vi "SentinelController v35 good v11.vi"() -> ()   [LabVIEW 2011] (continued)
                                n794 = Concatenate Strings(w2879, w2880, w2890, "   " ("string"), w2891, w2880, "H1 Warning, H2 Alarming", w2880, w2899, w2880, "H1 Low Yield Warning Limit: ", w2901, ", H1 yield = ", w2903, w2880, "H1 Low UPH Warning Limit: ", w2905, ", H1 UPH = ", w2907, w2880, w2908, w2880, "H2 Low Yield Alarm Limit: ", w2910, ", H2 yield = ", w2912, w2880, "H2 Low UPH Alarm Limit: ", w2914, ", H2 UPH = ", w2916, w2880, w2880) -> (w2888:string)
                                n795 = call "SentinelDatalog.vi"("operation (0:open)"=T10."open", "String"=w2888, "data log path"=w2882) -> ()  [unwired: 8 in, 1 out]
                                }
                                frame "H1AH2N" {
                                w2927 = "\r\n"
                                n796 = local read "H1 online"() -> (w2944:bool)
                                n797 = local read "H2 online"() -> (w2945:bool)
                                n798 = local read "H2 UPH warning limit hid"() -> (w2942:dbl)
                                n799 = local read "H2  low yield warning"() -> (w2941:dbl)
                                n800 = local read "H1 UPH alarm limit hid"() -> (w2940:dbl)
                                n801 = local read "H1 low yield alarm"() -> (w2939:dbl)
                                n802 = local read "H1 UPH"() -> (w2933:cluster{u32, u32})
                                n803 = local read "H2 UPH"() -> (w2932:cluster{u32, u32})
                                n804 = local read "YieldMon"() -> (w2925:cluster{i32, i32, i32, i32})
                                n805 = local read "YieldMon"() -> (w2923:cluster{i32, i32, i32, i32})
                                n806 = case shown="True" w2944 {
                                tunnel: ["H1 Off-Line" "H1 On-Line"] -> w2946
                                frame False {
                                }
                                frame True {
                                }
                                }
                                n807 = case shown="False" w2945 {
                                tunnel: ["H2 Off-Line" "H2 On-Line"] -> w2955
                                frame False {
                                }
                                frame True {
                                }
                                }
                                n808 = local read "Number of data log entries hid"() -> (w2921:u32)
                                n809 = Unbundle(w2925) -> (w2924:i32)  [unwired: 3 out]
                                n810 = Unbundle(w2933) -> (w2931:u32)  [unwired: 1 out]
                                n811 = Unbundle(w2923) -> (w2922:i32)  [unwired: 3 out]
                                n812 = Unbundle(w2932) -> (w2930:u32)  [unwired: 1 out]
                                n813 = Number To Decimal String(number=w2939) -> (decimal integer string=w2948:string)  [unwired: 1 in]
                                n814 = Number To Decimal String(number=w2924) -> (decimal integer string=w2950:string)  [unwired: 1 in]
                                n815 = Number To Decimal String(number=w2940) -> (decimal integer string=w2952:string)  [unwired: 1 in]
                                n816 = Number To Decimal String(number=w2931) -> (decimal integer string=w2954:string)  [unwired: 1 in]
                                n817 = Number To Decimal String(number=w2941) -> (decimal integer string=w2957:string)  [unwired: 1 in]
                                n818 = Number To Decimal String(number=w2922) -> (decimal integer string=w2959:string)  [unwired: 1 in]
                                n819 = Number To Decimal String(number=w2942) -> (decimal integer string=w2961:string)  [unwired: 1 in]
                                n820 = Number To Decimal String(number=w2930) -> (decimal integer string=w2963:string)  [unwired: 1 in]
                                n821 = local read "Data log path and filename"() -> (w2929:path)
                                n822 = Get Date/Time String(want seconds? (F)=TRUE) -> (date string=w2937:string, time string=w2938:string)  [unwired: 2 in]
                                n823 = Number To Decimal String(number=w2921) -> (decimal integer string=w2926:string)  [unwired: 1 in]
                                n824 = Concatenate Strings(w2926, w2927, w2937, "   " ("string"), w2938, w2927, "H1 Alarming, H2 Nominal", w2927, w2946, w2927, "H1 Low Yield Alarm Limit: ", w2948, ", H1 yield = ", w2950, w2927, "H1 Low UPH Alarm Limit: ", w2952, ", H1 UPH = ", w2954, w2927, w2955, w2927, "H2 Low Yield Warning Limit: ", w2957, ", H2 yield = ", w2959, w2927, "H2 Low UPH Warning Limit: ", w2961, ", H2 UPH = ", w2963, w2927, w2927) -> (w2935:string)
                                n825 = call "SentinelDatalog.vi"("operation (0:open)"=T10."open", "String"=w2935, "data log path"=w2929) -> ()  [unwired: 8 in, 1 out]
                                }
                                frame "H1AH2W" {
                                w2974 = "\r\n"
                                n826 = local read "H1 online"() -> (w2991:bool)
                                n827 = local read "H2 online"() -> (w2992:bool)
                                n828 = local read "H2 UPH warning limit hid"() -> (w2989:dbl)
                                n829 = local read "H2  low yield warning"() -> (w2988:dbl)
                                n830 = local read "H1 UPH alarm limit hid"() -> (w2987:dbl)
                                n831 = local read "H1 low yield alarm"() -> (w2986:dbl)
                                n832 = local read "H1 UPH"() -> (w2980:cluster{u32, u32})
                                n833 = local read "H2 UPH"() -> (w2979:cluster{u32, u32})
                                n834 = local read "YieldMon"() -> (w2972:cluster{i32, i32, i32, i32})
                                n835 = local read "YieldMon"() -> (w2970:cluster{i32, i32, i32, i32})
                                n836 = case shown="True" w2991 {
                                tunnel: ["H1 Off-Line" "H1 On-Line"] -> w2993
                                frame False {
                                }
                                frame True {
                                }
                                }
                                n837 = case shown="True" w2992 {
                                tunnel: ["H2 Off-Line" "H2 On-Line"] -> w3002
                                frame False {
                                }
                                frame True {
                                }
                                }
                                n838 = local read "Number of data log entries hid"() -> (w2968:u32)
                                n839 = Unbundle(w2972) -> (w2971:i32)  [unwired: 3 out]
                                n840 = Unbundle(w2980) -> (w2978:u32)  [unwired: 1 out]
                                n841 = Unbundle(w2970) -> (w2969:i32)  [unwired: 3 out]
                                n842 = Unbundle(w2979) -> (w2977:u32)  [unwired: 1 out]
                                n843 = Number To Decimal String(number=w2986) -> (decimal integer string=w2995:string)  [unwired: 1 in]
                                n844 = Number To Decimal String(number=w2971) -> (decimal integer string=w2997:string)  [unwired: 1 in]
                                n845 = Number To Decimal String(number=w2987) -> (decimal integer string=w2999:string)  [unwired: 1 in]
                                n846 = Number To Decimal String(number=w2978) -> (decimal integer string=w3001:string)  [unwired: 1 in]
                                n847 = Number To Decimal String(number=w2988) -> (decimal integer string=w3004:string)  [unwired: 1 in]
                                n848 = Number To Decimal String(number=w2969) -> (decimal integer string=w3006:string)  [unwired: 1 in]
                                n849 = Number To Decimal String(number=w2989) -> (decimal integer string=w3008:string)  [unwired: 1 in]
                                n850 = Number To Decimal String(number=w2977) -> (decimal integer string=w3010:string)  [unwired: 1 in]
                                n851 = local read "Data log path and filename"() -> (w2976:path)
                                n852 = Get Date/Time String(want seconds? (F)=TRUE) -> (date string=w2984:string, time string=w2985:string)  [unwired: 2 in]
                                n853 = Number To Decimal String(number=w2968) -> (decimal integer string=w2973:string)  [unwired: 1 in]
                                n854 = Concatenate Strings(w2973, w2974, w2984, "   " ("string"), w2985, w2974, "H1 Alarming, H2 Warning", w2974, w2993, w2974, "H1 Low Yield Alarm Limit: ", w2995, ", H1 yield = ", w2997, w2974, "H1 Low UPH Alarm Limit: ", w2999, ", H1 UPH = ", w3001, w2974, w3002, w2974, "H2 Low Yield Warning Limit: ", w3004, ", H2 yield = ", w3006, w2974, "H2 Low UPH Warning Limit: ", w3008, ", H2 UPH = ", w3010, w2974) -> (w2982:string)
                                n855 = call "SentinelDatalog.vi"("operation (0:open)"=T10."open", "String"=w2982, "data log path"=w2976) -> ()  [unwired: 8 in, 1 out]
                                }
                                frame "H1AH2A" {
                                w3021 = "\r\n"
                                n856 = local read "H1 online"() -> (w3038:bool)
                                n857 = local read "H2 online"() -> (w3039:bool)
                                n858 = local read "H1 UPH alarm limit hid"() -> (w3034:dbl)
                                n859 = local read "H2 UPH alarm limit hid"() -> (w3036:dbl)
                                n860 = local read "H1 low yield alarm"() -> (w3033:dbl)
                                n861 = local read "H1 UPH"() -> (w3027:cluster{u32, u32})
                                n862 = local read "H2 low yield alarm"() -> (w3035:dbl)
                                n863 = local read "H2 UPH"() -> (w3026:cluster{u32, u32})
                                n864 = local read "YieldMon"() -> (w3019:cluster{i32, i32, i32, i32})
                                n865 = local read "YieldMon"() -> (w3018:cluster{i32, i32, i32, i32})
                                n866 = case shown="True" w3038 {
                                tunnel: ["H1 Off-Line" "H1 On-Line"] -> w3040
                                frame False {
                                }
                                frame True {
                                }
                                }
                                n867 = case shown="True" w3039 {
                                tunnel: ["H2 Off-Line" "H2 On-Line"] -> w3049
                                frame False {
                                }
                                frame True {
                                }
                                }
                                n868 = local read "Number of data log entries hid"() -> (w3015:u32)
                                n869 = Unbundle(w3019) -> (w3016:i32)  [unwired: 3 out]
                                n870 = Unbundle(w3027) -> (w3025:u32)  [unwired: 1 out]
                                n871 = Unbundle(w3018) -> (w3017:i32)  [unwired: 3 out]
                                n872 = Unbundle(w3026) -> (w3024:u32)  [unwired: 1 out]
                                n873 = Number To Decimal String(number=w3033) -> (decimal integer string=w3042:string)  [unwired: 1 in]
                                n874 = Number To Decimal String(number=w3016) -> (decimal integer string=w3044:string)  [unwired: 1 in]
                                n875 = Number To Decimal String(number=w3034) -> (decimal integer string=w3046:string)  [unwired: 1 in]
                                n876 = Number To Decimal String(number=w3025) -> (decimal integer string=w3048:string)  [unwired: 1 in]
                                n877 = Number To Decimal String(number=w3035) -> (decimal integer string=w3051:string)  [unwired: 1 in]
                                n878 = Number To Decimal String(number=w3017) -> (decimal integer string=w3053:string)  [unwired: 1 in]
                                n879 = Number To Decimal String(number=w3036) -> (decimal integer string=w3055:string)  [unwired: 1 in]
                                n880 = Number To Decimal String(number=w3024) -> (decimal integer string=w3057:string)  [unwired: 1 in]
                                n881 = local read "Data log path and filename"() -> (w3023:path)
                                n882 = Get Date/Time String(want seconds? (F)=TRUE) -> (date string=w3031:string, time string=w3032:string)  [unwired: 2 in]
                                n883 = Number To Decimal String(number=w3015) -> (decimal integer string=w3020:string)  [unwired: 1 in]
                                n884 = Concatenate Strings(w3020, w3021, w3031, "   " ("string"), w3032, w3021, "H1 Alarming, H2 Alarming", w3021, w3040, w3021, "H1 Low Yield Alarm Limit: ", w3042, ", H1 yield = ", w3044, w3021, "H1 Low UPH Alarm Limit: ", w3046, ", H1 UPH = ", w3048, w3021, w3049, w3021, "H2 Low Yield Alarm Limit: ", w3051, ", H2 yield = ", w3053, w3021, "H2 Low UPH Alarm Limit: ", w3055, ", H2 UPH = ", w3057, w3021, w3021) -> (w3029:string)
                                n885 = call "SentinelDatalog.vi"("operation (0:open)"=T10."open", "String"=w3029, "data log path"=w3023) -> ()  [unwired: 8 in, 1 out]
                                }
                                }
                                }
                                frame #2 {
                                n886 = Wait (ms)(milliseconds to wait=u32 100) -> ()  [unwired: 1 out]
                                }
                                frame #3 {
                                n887 = local read "Enable electronic notification of alarms"() -> (w3063:bool)
                                n888 = case shown="True" w3063 {
                                frame False {
                                }
                                frame True {
                                n889 = stacked-sequence {
                                frame #0 {
                                # "Email"
                                n890 = local read "Enable email notification"() -> (w3066:bool)
                                n891 = local read "Number of email alerts"() -> (w3065:u32)
                                n892 = Increment(x=w3065) -> (x+1=w3064:u32)
                                n893 = local write "Number of email alerts"(w3064) -> ()
                                n894 = case shown="True" w3066 {
                                frame False {
                                }
                                frame True {
                                n895 = flat-sequence {
                                tunnel: [w3073] -> w3068
                                tunnel: [w3081] -> w3067
                                tunnel: w3068 -> [w3081]
                                tunnel: w3067 -> [w3082]
                                frame #0 {
                                n896 = local read "Data log path and filename"() -> (w3078:path)
                                n897 = local read "Number of email alerts"() -> (w3072:u32)
                                n898 = Number To Decimal String(number=w3072) -> (decimal integer string=w3071:string)  [unwired: 1 in]
                                n899 = Strip Path(path=w3078) -> (stripped path=w3076:path, name=w3070:string)
                                n900 = Path To String(path=w3076) -> (string=w3075:string)
                                n901 = Concatenate Strings(w3075, "\\sent_#" ("string"), w3071, "_" ("string"), w3070) -> (w3079:string)
                                n902 = String To Path(string=w3079) -> (path=w3074:path)
                                n903 = Copy(10:w3074, 11:w3078) -> (3:w3073:path)  [unwired: 3 in, 2 out]
                                }
                                frame #1 {
                                n904 = Wait (ms)(milliseconds to wait=u32 1000) -> ()  [unwired: 1 out]
                                }
                                frame #2 {
                                n905 = local read "Email alert - engineer"() -> (w3084:string)
                                n906 = local read "Email alert - CC"() -> (w3083:string)
                                n907 = local read "Email alert - message"() -> (w3085:string)
                                n908 = call "email_alert.vi"("Email Alert - Message"=w3085, "Email Alert - Engineer"=w3084, "Email Alert - CC"=w3083, "Email ALert - Attachment"=w3082) -> ()  [unwired: 8 in]
                                }
                                }
                                }
                                }
                                }
                                frame #1 {
                                n909 = Wait (ms)(milliseconds to wait=u32 200) -> ()  [unwired: 1 out]
                                }
                                frame #2 {
                                # "text"
                                n910 = local read "Enable text notification"() -> (w3087:bool)
                                n911 = case shown="True" w3087 {
                                frame False {
                                }
                                frame True {
                                n912 = local read "Number of text alerts"() -> (w3091:u32)
                                n913 = Increment(x=w3091) -> (x+1=w3090:u32)
                                n914 = local write "Number of text alerts"(w3090) -> ()
                                n915 = local read "Number of email alerts"() -> (w3100:u32)
                                n916 = local read "Carrier"() -> (w3093:enum16{"T-Mobile", "AT&T", "Verizon", "Sprint"})
                                n917 = local read "Phone number"() -> (w3092:string)
                                n918 = local read "Body"() -> (w3089:string)
                                n919 = local read "Lot number"() -> (w3094:string)
                                n920 = local read "Subject"() -> (w3088:string)
                                n921 = Number To Decimal String(number=w3100) -> (decimal integer string=w3096:string)  [unwired: 1 in]
                                n922 = Concatenate Strings(w3089, ", # " ("string"), w3096, ", Lot Number: " ("string"), w3094) -> (w3101:string)
                                n923 = local write "Notifications Lot Display"(w3094) -> ()
                                n924 = call <userlib>:"Send SMS 2009.vi"("Body"=w3101, "Carrier"=w3093, "Subject"=w3088, "phone number"=w3092, "smtp server"="smtp.gmail.com", "password"="sentinelcontroller", "email username"="sentinelcontroller@gmail.com") -> ("Error Out"=w3099:errorcluster)  [unwired: 4 in]
                                n925 = Unbundle By Name(w3099) -> ("status"=w3098:bool)
                                n926 = case shown="True" w3098 {
                                frame False {
                                }
                                frame True {
                                n927 = One Button Dialog(message="Warning:\nError sending text message!\nTry changing the settings or\nswitch to email method", button name ("OK")="Dismiss") -> ()  [unwired: 1 out]
                                }
                                }
                                }
                                }
                                }
                                }
                                }
                                }
                                }
                                frame #4 {
                                n928 = Wait (ms)(milliseconds to wait=u32 100) -> ()  [unwired: 1 out]
                                }
                              }
                            }
                          }
                        }
                      }
                    }
                  }
                }
              }
              n929 = Wait (ms)(milliseconds to wait=u32 100) -> ()  [unwired: 1 out]
            }
            n930 = local read "Yield averaging"() -> (w350:u32)
            n931 = local read "UPH averaging"() -> (w349:u32)
            n932 = local read "Yield averaging"() -> (w351:u32)
            n933 = local read "UPH averaging"() -> (w352:u32)
            n934 = Initialize Array(w347, w350) -> (w348:i32[])
            n935 = Initialize Array(w346, w349) -> (w345:dbl[])
            n936 = Initialize Array(w354, w351) -> (w353:i32[])
            n937 = Initialize Array(w355, w352) -> (w356:dbl[])
            n938 = while {
              shift-right: [w2370] -> _
              shift-left: w346 -> [w2376]
              shift-right: [w2371] -> _
              shift-left: w345 -> [w2375]
              shift-right: [w2372] -> _
              shift-left: w347 -> [w2369]
              shift-right: [w2373] -> _
              shift-left: w348 -> [w2374]
              stop <- w2367 stop-if-true
              # "if there is now a lock, it is unlikely that the test time is going to be less than 100ms,\nso this is a relatively slow loop"
              n939 = local read "H2 Lock"() -> (w2366:bool)
              n940 = Wait (ms)(milliseconds to wait=u32 50) -> ()  [unwired: 1 out]
              n941 = case shown="True" w2366 {
                tunnel: w2376 -> [w2381 w2406]
                tunnel: w2375 -> [w2380 w2401]
                tunnel: w2374 -> [w2378 w2398]
                tunnel: [w2378 w2392] -> w2373
                tunnel: [w2379 w2390] -> w2372
                tunnel: [w2380 w2389] -> w2371
                tunnel: [w2381 w2388] -> w2370
                tunnel: w2369 -> [w2379 w2387]
                frame False {
                  n942 = local write "Calc H1 UPH"(u32 0 ("Sim H1 UPH")) -> ()
                }
                frame True {
                  n943 = flat-sequence {
                    tunnel: w2398 -> [w2409]
                    tunnel: w2387 -> [w2410]
                    tunnel: w2401 -> [w2411]
                    tunnel: w2406 -> [w2412]
                    tunnel: [w2412] -> w2397
                    tunnel: [w2411] -> w2396
                    tunnel: [w2410] -> w2395
                    tunnel: [w2409] -> w2394
                    tunnel: [w2425] -> w2405
                    tunnel: [w2424] -> w2402
                    tunnel: [w2423] -> w2400
                    tunnel: [w2422] -> w2399
                    tunnel: w2397 -> [w2425]
                    tunnel: w2396 -> [w2424]
                    tunnel: w2395 -> [w2423]
                    tunnel: w2394 -> [w2422]
                    tunnel: w2405 -> [w2451]
                    tunnel: [w2451] -> w2404
                    tunnel: [w2450] -> w2403
                    tunnel: w2402 -> [w2450]
                    tunnel: w2400 -> [w2440]
                    tunnel: w2399 -> [w2439]
                    tunnel: [w2438] -> w2393
                    tunnel: [w2437] -> w2391
                    tunnel: w2404 -> [w2477]
                    tunnel: w2403 -> [w2478]
                    tunnel: w2393 -> [w2496]
                    tunnel: w2391 -> [w2495]
                    tunnel: [w2496] -> w2386
                    tunnel: [w2495] -> w2385
                    tunnel: [w2474] -> w2384
                    tunnel: [w2473] -> w2383
                    tunnel: [w2511] -> w2388
                    tunnel: [w2512] -> w2389
                    tunnel: [w2513] -> w2390
                    tunnel: [w2514] -> w2392
                    tunnel: w2386 -> [w2514]
                    tunnel: w2385 -> [w2513]
                    tunnel: w2384 -> [w2512]
                    tunnel: w2383 -> [w2511]
                    frame #0 {
                      n944 = local read "H2 loop counter hid"() -> (w2407:u32)
                      n945 = Equal To 0?(x=w2407) -> (x = 0?=w2408:bool)
                      n946 = case shown="True" w2408 {
                        frame False {
                        }
                        frame True {
                          # "H2 first pass init"
                          n947 = local write "H2 Device Count"(0.0 ("H2 Device Count")) -> ()
                          n948 = local write "H2 measured  Index Time"(0.0 ("H2 Index Time")) -> ()
                          n949 = local write "H2 measured Test Time"(0.0 ("H2 Test Time")) -> ()
                          n950 = local write "H2 measured Wait Time"(0.0 ("H2 Wait Time")) -> ()
                          n951 = local read "H2 low UPH alarm (%)"() -> (w2416:dbl)
                          n952 = Divide(x=w2416, y=100.0) -> (x/y=w2415:dbl)
                          n953 = Bundle(0.0, w2415) -> (w2413:cluster{dbl, dbl})  [unwired: 1 in]
                          n954 = local write "H2 UPH"(w2413) -> ()
                        }
                      }
                    }
                    frame #1 {
                      # "H2 testing"
                      n955 = while {
                        stop <- w2429 stop-if-true
                        n956 = local read "H2 Lock"() -> (w2433:bool)
                        n957 = local read "POWER"() -> (w2428:bool)
                        n958 = local read "Run"() -> (w2426:bool)
                        n959 = Not(x=w2433) -> (.not. x?=w2427:bool)
                        n960 = Not(x=w2428) -> (.not. x?=w2431:bool)
                        n961 = Not(x=w2426) -> (.not. x?=w2430:bool)
                        n962 = Compound Arithmetic op=OR(w2427, w2431, w2430) -> (w2429:bool)
                        n963 = Wait (ms)(milliseconds to wait=u32 1) -> ()  [unwired: 1 out]
                      }
                    }
                    frame #2 {
                      n964 = local read "H2 cycle yield hid"() -> (w2434:dbl)
                      n965 = local read "H2 loop counter hid"() -> (w2435:u32)
                      n966 = local read "Yield averaging"() -> (w2436:u32)
                      n967 = local read "H2 low yield alarm"() -> (w2449:dbl)
                      n968 = local read "YieldMon"() -> (w2442:cluster{i32, i32, i32, i32})
                      n969 = local read "H2  low yield warning"() -> (w2448:dbl)
                      n970 = call "moving_avg_core.vi"("Array in"=w2439, "avg"=w2436, "accumulator in"=w2440, "i"=w2435, "data in"=w2434) -> ("Array out"=w2438:dbl[], "accumulator out"=w2437:dbl, "rolling avg out"=w2443:dbl)  [unwired: 4 in]
                      n971 = Unbundle(w2442) -> (w2441:i32)  [unwired: 3 out]
                      n972 = Less?(x=w2443, y=w2448) -> (x < y?=w2447:bool)
                      n973 = case shown="True" w2447 {
                        tunnel: w2443 -> [_ w2456]
                        tunnel: w2449 -> [_ w2455]
                        frame False {
                          n974 = local write "H2 nominal"(TRUE ("H1 nominal")) -> ()
                          n975 = local write "H2 warning"(FALSE ("H1 warning")) -> ()
                          n976 = local write "H2 alarm"(FALSE ("H1 warning")) -> ()
                        }
                        frame True {
                          n977 = Less?(x=w2456, y=w2455) -> (x < y?=w2457:bool)
                          n978 = case shown="True" w2457 {
                            frame False {
                              n979 = local write "H2 nominal"(FALSE ("H1 nominal")) -> ()
                              n980 = local write "H2 warning"(TRUE ("H1 warning")) -> ()
                              n981 = local write "H2 alarm"(FALSE ("H1 warning")) -> ()
                            }
                            frame True {
                              n982 = local read "H2 enable halt\non yield alarm"() -> (w2461:bool)
                              n983 = local write "H2 nominal"(FALSE ("H1 nominal")) -> ()
                              n984 = local write "H2 alarm"(TRUE ("H1 warning")) -> ()
                              n985 = local write "H2 warning"(FALSE ("H1 warning")) -> ()
                              n986 = case shown="True" w2461 {
                                frame False {
                                }
                                frame True {
                                n987 = local write "H2 online"(FALSE ("H1 Online")) -> ()
                                }
                              }
                            }
                          }
                        }
                      }
                      n988 = local read "H1 low yield alarm"() -> (w2446:dbl)
                      n989 = local read "H2 low yield alarm"() -> (w2445:dbl)
                      n990 = Bundle(w2441, "rolling avg out"=w2443, "H1 low yield alarm"=w2446, "H2 low yield alarm"=w2445) -> (w2444:T12)  [unwired: 1 in]
                      n991 = local write "YieldMon"(w2444) -> ()
                    }
                    frame #3 {
                      n992 = local read "H2 measured  Index Time"() -> (w2467:dbl)
                      n993 = local read "H2 measured Wait Time"() -> (w2466:dbl)
                      n994 = local read "H2 measured Test Time"() -> (w2468:dbl)
                      n995 = local read "H2 parallelism"() -> (w2480:u32)
                      n996 = local read "H2 lot yield mon"() -> (w2494:dbl)
                      n997 = local write "H2 IT (scycle)"(w2467) -> ()
                      n998 = local write "H2 TT (s/cycle)"(w2468) -> ()
                      n999 = local write "H2 WT (s/cycle)"(w2466) -> ()
                      n1000 = Compound Arithmetic op=ADD(w2467, w2468, w2466) -> (w2483:dbl)
                      n1001 = Compound Arithmetic op=ADD(w2467, w2468) -> (w2479:dbl)
                      n1002 = Multiply(x=w2480, y=3600.0 ("x")) -> (x*y=w2482:dbl)
                      n1003 = Divide(x=w2482, y=w2483) -> (x/y=w2493:dbl)
                      n1004 = Divide(x=w2494, y=w2479) -> (x/y=w2472:dbl)
                      n1005 = local write "H2 Single Handler UPH hid"(w2472) -> ()
                      n1006 = local read "H2 low UPH warning (%)"() -> (w2490:dbl)
                      n1007 = local read "H2 loop counter hid"() -> (w2476:u32)
                      n1008 = local read "Yield averaging"() -> (w2475:u32)
                      n1009 = local read "H2 low UPH alarm (%)"() -> (w2485:dbl)
                      n1010 = property on="H2 UPH" class="Knob (strict)"() -> ("Scale.Maximum"=w2491:dbl)  [unwired: 2 in, 2 out]
                      n1011 = Divide(x=w2490, y=100.0) -> (x/y=w2489:dbl)
                      n1012 = call "moving_avg_core.vi"("Array in"=w2478, "avg"=w2475, "accumulator in"=w2477, "i"=w2476, "data in"=w2493) -> ("Array out"=w2474:dbl[], "accumulator out"=w2473:dbl, "rolling avg out"=w2492:dbl)  [unwired: 4 in]
                      n1013 = Multiply(x=w2491, y=w2489) -> (x*y=w2471:dbl)
                      n1014 = Divide(x=w2485, y=100.0) -> (x/y=w2487:dbl)
                      n1015 = local write "H2 UPH warning limit hid"(w2471) -> ()
                      n1016 = Less?(x=w2492, y=w2471) -> (x < y?=w2484:bool)
                      n1017 = Multiply(x=w2491, y=w2487) -> (x*y=w2470:dbl)
                      n1018 = case shown="True" w2484 {
                        tunnel: w2492 -> [_ w2501]
                        tunnel: w2470 -> [_ w2500]
                        frame False {
                          n1019 = local write "H2 nominal 2"(TRUE ("H1 nominal")) -> ()
                          n1020 = local write "H2 warning 2"(FALSE ("H1 warning")) -> ()
                          n1021 = local write "H2 alarm 2"(FALSE ("H1 warning")) -> ()
                        }
                        frame True {
                          n1022 = Less?(x=w2501, y=w2500) -> (x < y?=w2502:bool)
                          n1023 = case shown="True" w2502 {
                            frame False {
                              n1024 = local write "H2 nominal 2"(FALSE ("H1 nominal")) -> ()
                              n1025 = local write "H2 warning 2"(TRUE ("H1 warning")) -> ()
                              n1026 = local write "H2 alarm 2"(FALSE ("H1 warning")) -> ()
                            }
                            frame True {
                              n1027 = local read "H2 enable halt\non UPH alarm"() -> (w2506:bool)
                              n1028 = local write "H2 alarm 2"(TRUE ("H1 warning")) -> ()
                              n1029 = local write "H2 warning 2"(FALSE ("H1 warning")) -> ()
                              n1030 = local write "H2 nominal 2"(FALSE ("H1 nominal")) -> ()
                              n1031 = case shown="True" w2506 {
                                frame False {
                                }
                                frame True {
                                n1032 = local write "H2 online"(FALSE ("H1 Online")) -> ()
                                }
                              }
                            }
                          }
                        }
                      }
                      n1033 = local write "H2 UPH alarm limit hid"(w2470) -> ()
                      n1034 = Bundle("rolling avg out"=w2492, w2470) -> (w2469:cluster{"rolling avg out":dbl, dbl})  [unwired: 1 in]
                      n1035 = local write "H2 UPH"(w2469) -> ()
                    }
                    frame #4 {
                      n1036 = while {
                        stop <- w2516 continue-if-true
                        n1037 = local read "H2 Lock"() -> (w2516:bool)
                        n1038 = Wait (ms)(milliseconds to wait=u32 10) -> ()  [unwired: 1 out]
                      }
                    }
                  }
                }
              }
              n1039 = local read "POWER"() -> (w2368:bool)
              n1040 = Not(x=w2368) -> (.not. x?=w2367:bool)
            }
            n1041 = while {
              shift-right: [w3247] -> _
              shift-left: w355 -> [w3250]
              shift-right: [w3248] -> _
              shift-left: w356 -> [w3249]
              shift-right: [w3243] -> _
              shift-left: w354 -> [w3246]
              shift-right: [w3244] -> _
              shift-left: w353 -> [w3245]
              stop <- w3242 stop-if-true
              # "if there is now a lock, it is unlikely that the test time is going to be less than 100ms,\nso this is a relatively slow loop"
              n1042 = local read "H1 Lock"() -> (w3241:bool)
              n1043 = case shown="True" w3241 {
                tunnel: w3250 -> [w3256 w3281]
                tunnel: w3249 -> [w3255 w3276]
                tunnel: [w3255 w3275] -> w3248
                tunnel: [w3256 w3274] -> w3247
                tunnel: w3246 -> [w3254 w3272]
                tunnel: w3245 -> [w3253 w3270]
                tunnel: [w3253 w3268] -> w3244
                tunnel: [w3254 w3266] -> w3243
                frame False {
                  n1044 = local write "Calc H1 UPH"(u32 0 ("Sim H1 UPH")) -> ()
                }
                frame True {
                  n1045 = flat-sequence {
                    tunnel: w3270 -> [w3284]
                    tunnel: w3272 -> [w3285]
                    tunnel: w3276 -> [w3286]
                    tunnel: w3281 -> [w3287]
                    tunnel: [w3287] -> w3265
                    tunnel: [w3286] -> w3264
                    tunnel: [w3285] -> w3263
                    tunnel: [w3284] -> w3262
                    tunnel: [w3300] -> w3280
                    tunnel: [w3299] -> w3277
                    tunnel: [w3298] -> w3273
                    tunnel: [w3297] -> w3271
                    tunnel: w3265 -> [w3300]
                    tunnel: w3264 -> [w3299]
                    tunnel: w3263 -> [w3298]
                    tunnel: w3262 -> [w3297]
                    tunnel: w3280 -> [w3315]
                    tunnel: [w3315] -> w3279
                    tunnel: [w3314] -> w3278
                    tunnel: w3277 -> [w3314]
                    tunnel: w3273 -> [w3313]
                    tunnel: w3271 -> [w3312]
                    tunnel: [w3311] -> w3269
                    tunnel: [w3310] -> w3267
                    tunnel: w3279 -> [w3353]
                    tunnel: w3278 -> [w3352]
                    tunnel: w3269 -> [w3349]
                    tunnel: w3267 -> [w3348]
                    tunnel: [w3351] -> w3261
                    tunnel: [w3350] -> w3260
                    tunnel: [w3349] -> w3259
                    tunnel: [w3348] -> w3258
                    tunnel: [w3388] -> w3266
                    tunnel: [w3389] -> w3268
                    tunnel: [w3390] -> w3274
                    tunnel: [w3391] -> w3275
                    tunnel: w3261 -> [w3391]
                    tunnel: w3260 -> [w3390]
                    tunnel: w3259 -> [w3389]
                    tunnel: w3258 -> [w3388]
                    frame #0 {
                      n1046 = local read "H1 loop counter hid"() -> (w3283:u32)
                      n1047 = Equal To 0?(x=w3283) -> (x = 0?=w3282:bool)
                      n1048 = case shown="True" w3282 {
                        frame False {
                        }
                        frame True {
                          n1049 = local read "H1 low UPH alarm (%)"() -> (w3292:dbl)
                          n1050 = local write "H1 measured Index Time"(0.0 ("H1 Index Time")) -> ()
                          n1051 = local write "H1 measured Wait Time"(0.0 ("H1 Wait Time")) -> ()
                          n1052 = local write "H1 Device Count"(0.0 ("H1 Device Count")) -> ()
                          n1053 = local write "H1 measured Test Time"(0.0 ("H1 Test Time")) -> ()
                          n1054 = Divide(x=w3292, y=100.0) -> (x/y=w3290:dbl)
                          n1055 = Bundle("y"=0.0, w3290) -> (w3288:cluster{"y":dbl, dbl})  [unwired: 1 in]
                          n1056 = local write "H1 UPH"(w3288) -> ()
                        }
                      }
                    }
                    frame #1 {
                      # "H1 testing"
                      n1057 = while {
                        stop <- w3304 stop-if-true
                        n1058 = local read "H1 Lock"() -> (w3308:bool)
                        n1059 = local read "POWER"() -> (w3302:bool)
                        n1060 = local read "Run"() -> (w3301:bool)
                        n1061 = Wait (ms)(milliseconds to wait=u32 1) -> ()  [unwired: 1 out]
                        n1062 = Not(x=w3308) -> (.not. x?=w3303:bool)
                        n1063 = Not(x=w3302) -> (.not. x?=w3306:bool)
                        n1064 = Not(x=w3301) -> (.not. x?=w3305:bool)
                        n1065 = Compound Arithmetic op=OR(w3303, w3306, w3305) -> (w3304:bool)
                      }
                    }
                    frame #2 {
                      n1066 = local read "H1 cycle yield hid"() -> (w3318:dbl)
                      n1067 = local read "H1 loop counter hid"() -> (w3317:u32)
                      n1068 = local read "Yield averaging"() -> (w3316:u32)
                      n1069 = local read "H1 low yield warning"() -> (w3326:dbl)
                      n1070 = local read "H1 low yield alarm"() -> (w3324:dbl)
                      n1071 = call "moving_avg_core.vi"("Array in"=w3312, "avg"=w3316, "accumulator in"=w3313, "i"=w3317, "data in"=w3318) -> ("Array out"=w3311:dbl[], "accumulator out"=w3310:dbl, "rolling avg out"=w3321:dbl)  [unwired: 4 in]
                      n1072 = Less?(x=w3321, y=w3326) -> (x < y?=w3325:bool)
                      n1073 = case shown="True" w3325 {
                        tunnel: w3321 -> [_ w3332]
                        tunnel: w3324 -> [_ w3331]
                        frame False {
                          n1074 = local write "H1 alarm"(FALSE ("H1 warning")) -> ()
                          n1075 = local write "H1 warning"(FALSE ("H1 warning")) -> ()
                          n1076 = local write "H1 nominal"(TRUE ("H1 nominal")) -> ()
                        }
                        frame True {
                          n1077 = Less?(x=w3332, y=w3331) -> (x < y?=w3330:bool)
                          n1078 = case shown="True" w3330 {
                            frame False {
                              n1079 = local write "H1 alarm"(FALSE ("H1 warning")) -> ()
                              n1080 = local write "H1 warning"(TRUE ("H1 warning")) -> ()
                              n1081 = local write "H1 nominal"(FALSE ("H1 nominal")) -> ()
                            }
                            frame True {
                              n1082 = local read "H1 enable halt\non yield alarm"() -> (w3336:bool)
                              n1083 = local write "H1 nominal"(FALSE ("H1 nominal")) -> ()
                              n1084 = local write "H1 warning"(FALSE ("H1 warning")) -> ()
                              n1085 = local write "H1 alarm"(TRUE ("H1 warning")) -> ()
                              n1086 = case shown="True" w3336 {
                                frame False {
                                }
                                frame True {
                                n1087 = local write "H1 online"(FALSE ("H1 Online")) -> ()
                                }
                              }
                            }
                          }
                        }
                      }
                      n1088 = local read "YieldMon"() -> (w3320:cluster{i32, i32, i32, i32})
                      n1089 = local read "H1 low yield alarm"() -> (w3323:dbl)
                      n1090 = local read "H2 low yield alarm"() -> (w3322:dbl)
                      n1091 = Unbundle(w3320) -> (w3309:i32)  [unwired: 3 out]
                      n1092 = Bundle("rolling avg out"=w3321, w3309, "H1 low yield alarm"=w3323, "H2 low yield alarm"=w3322) -> (w3319:T13)  [unwired: 1 in]
                      n1093 = local write "YieldMon"(w3319) -> ()
                    }
                    frame #3 {
                      n1094 = local read "H1 measured Index Time"() -> (w3343:dbl)
                      n1095 = local read "H1 measured Wait Time"() -> (w3341:dbl)
                      n1096 = local read "H1 measured Test Time"() -> (w3342:dbl)
                      n1097 = local read "H1 parallelism"() -> (w3360:u32)
                      n1098 = local read "H1 loop counter hid"() -> (w3355:u32)
                      n1099 = local read "UPH averaging"() -> (w3354:u32)
                      n1100 = local read "H1 low UPH warning (%)"() -> (w3364:dbl)
                      n1101 = local write "H1 IT (s/cycle)"(w3343) -> ()
                      n1102 = local write "H1 TT (s/cycle)"(w3342) -> ()
                      n1103 = local write "H1 WT (s/cycle)"(w3341) -> ()
                      n1104 = Compound Arithmetic op=ADD(w3343, w3342, w3341) -> (w3356:dbl)
                      n1105 = Compound Arithmetic op=ADD(w3343, w3342) -> (w3363:dbl)
                      n1106 = Multiply(x=w3360, y=u32 3600 ("x")) -> (x*y=w3362:u32)
                      n1107 = Divide(x=w3362, y=w3363) -> (x/y=w3346:dbl)
                      n1108 = local read "H1 low UPH alarm (%)"() -> (w3369:dbl)
                      n1109 = local write "H1 Single Handler UPH hid"(w3346) -> ()
                      n1110 = property on="H1 UPH" class="Knob (strict)"() -> ("Scale.Maximum"=w3371:dbl)  [unwired: 2 in, 2 out]
                      n1111 = Divide(x=w3364, y=100.0) -> (x/y=w3365:dbl)
                      n1112 = Multiply(x=w3371, y=w3365) -> (x*y=w3344:dbl)
                      n1113 = Divide(x=w3369, y=100.0) -> (x/y=w3367:dbl)
                      n1114 = local write "H1 UPH warning limit hid"(w3344) -> ()
                      n1115 = Multiply(x=w3371, y=w3367) -> (x*y=w3345:dbl)
                      n1116 = local write "H1 UPH alarm limit hid"(w3345) -> ()
                      n1117 = local read "H1 parallelism"() -> (w3359:u32)
                      n1118 = Multiply(x=w3359, y=u32 3600 ("x")) -> (x*y=w3357:u32)
                      n1119 = Divide(x=w3357, y=w3356) -> (x/y=w3373:dbl)
                      n1120 = call "moving_avg_core.vi"("Array in"=w3352, "avg"=w3354, "accumulator in"=w3353, "i"=w3355, "data in"=w3373) -> ("Array out"=w3351:dbl[], "accumulator out"=w3350:dbl, "rolling avg out"=w3372:dbl)  [unwired: 4 in]
                      n1121 = Less?(x=w3372, y=w3344) -> (x < y?=w3370:bool)
                      n1122 = case shown="True" w3370 {
                        tunnel: w3372 -> [_ w3378]
                        tunnel: w3345 -> [_ w3377]
                        frame False {
                          n1123 = local write "H1 alarm 2"(FALSE ("H1 warning")) -> ()
                          n1124 = local write "H1 nominal 2"(TRUE ("H1 nominal")) -> ()
                          n1125 = local write "H1 warning 2"(FALSE ("H1 warning")) -> ()
                        }
                        frame True {
                          n1126 = Less?(x=w3378, y=w3377) -> (x < y?=w3379:bool)
                          n1127 = case shown="True" w3379 {
                            frame False {
                              n1128 = local write "H1 nominal 2"(FALSE ("H1 nominal")) -> ()
                              n1129 = local write "H1 warning 2"(TRUE ("H1 warning")) -> ()
                              n1130 = local write "H1 alarm 2"(FALSE ("H1 warning")) -> ()
                            }
                            frame True {
                              n1131 = local read "H1 enable halt\non UPH alarm"() -> (w3383:bool)
                              n1132 = local write "H1 warning 2"(FALSE ("H1 warning")) -> ()
                              n1133 = local write "H1 alarm 2"(TRUE ("H1 warning")) -> ()
                              n1134 = local write "H1 nominal 2"(FALSE ("H1 nominal")) -> ()
                              n1135 = case shown="True" w3383 {
                                frame False {
                                }
                                frame True {
                                n1136 = local write "H1 online"(FALSE ("H1 Online")) -> ()
                                }
                              }
                            }
                          }
                        }
                      }
                      n1137 = Bundle("rolling avg out"=w3372, w3345) -> (w3347:cluster{"rolling avg out":dbl, dbl})  [unwired: 1 in]
                      n1138 = local write "H1 UPH"(w3347) -> ()
                    }
                    frame #4 {
                      n1139 = while {
                        stop <- w3393 continue-if-true
                        n1140 = local read "H1 Lock"() -> (w3393:bool)
                        n1141 = Wait (ms)(milliseconds to wait=u32 10) -> ()  [unwired: 1 out]
                      }
                    }
                  }
                }
              }
              n1142 = Wait (ms)(milliseconds to wait=u32 50) -> ()  [unwired: 1 out]
              n1143 = local read "POWER"() -> (w3252:bool)
              n1144 = Not(x=w3252) -> (.not. x?=w3242:bool)
            }
            n1145 = while {
              stop <- w932 continue-if-true
              n1146 = while {
                stop <- w934 stop-if-true
                n1147 = event shown="[1] \"H1 online\": Value Change" {
                  selector: _ -> [_ _]
                  dyn-events: _ -> [_ _]
                  timeout: -1 -> [_ _]
                  tunnel: [_ TRUE] -> w934
                  event Timeout {
                    n1148 = event-data() -> ()  [unwired: 1 in, 2 out]
                  }
                  event "H1 online": Value Change {
                    n1149 = event-data() -> ()  [unwired: 1 in, 5 out]
                    n1150 = local read "Enable data logging of all events"() -> (w935:bool)
                    n1151 = case shown="True" w935 {
                      frame False {
                      }
                      frame True {
                        w939 = "\r\n"
                        n1152 = Get Date/Time String(want seconds? (F)=TRUE) -> (date string=w944:string, time string=w943:string)  [unwired: 2 in]
                        n1153 = local read "H1 online"() -> (w941:bool)
                        n1154 = case shown="False" w941 {
                          tunnel: ["H1 Off-Line" "H1 On-Line"] -> w940
                          frame False {
                          }
                          frame True {
                          }
                        }
                        n1155 = local read "Data log path and filename"() -> (w938:path)
                        n1156 = Concatenate Strings(w944, "   " ("string"), w943, w939, "Change in H1 Status: ", w940, w939, w939) -> (w946:string)
                        n1157 = call "SentinelDatalog.vi"("operation (0:open)"=T10."open", "String"=w946, "data log path"=w938) -> ()  [unwired: 8 in, 1 out]
                      }
                    }
                  }
                }
              }
              n1158 = local read "POWER"() -> (w932:bool)
            }
            n1159 = while {
              stop <- w914 continue-if-true
              n1160 = while {
                stop <- w916 stop-if-true
                n1161 = event shown="[1] \"H2 online\": Value Change" {
                  selector: _ -> [_ _]
                  dyn-events: _ -> [_ _]
                  timeout: -1 -> [_ _]
                  tunnel: [_ TRUE] -> w916
                  event Timeout {
                    n1162 = event-data() -> ()  [unwired: 1 in, 2 out]
                  }
                  event "H2 online": Value Change {
                    n1163 = event-data() -> ()  [unwired: 1 in, 5 out]
                    n1164 = local read "Enable data logging of all events"() -> (w917:bool)
                    n1165 = case shown="True" w917 {
                      frame False {
                      }
                      frame True {
                        w921 = "\r\n"
                        n1166 = local read "H2 online"() -> (w923:bool)
                        n1167 = case shown="False" w923 {
                          tunnel: ["H2 Off-Line" "H2 On-Line"] -> w922
                          frame False {
                          }
                          frame True {
                          }
                        }
                        n1168 = local read "Data log path and filename"() -> (w920:path)
                        n1169 = Get Date/Time String(want seconds? (F)=TRUE) -> (date string=w926:string, time string=w925:string)  [unwired: 2 in]
                        n1170 = Concatenate Strings(w926, "   " ("string"), w925, w921, "Change in H2 Status: ", w922, w921, w921) -> (w928:string)
                        n1171 = call "SentinelDatalog.vi"("operation (0:open)"=T10."open", "String"=w928, "data log path"=w920) -> ()  [unwired: 8 in, 1 out]
                      }
                    }
                  }
                }
              }
              n1172 = local read "POWER"() -> (w914:bool)
            }
            n1173 = while {
              stop <- w1062 continue-if-true
              n1174 = local read "Tester online"() -> (w1063:bool)
              n1175 = case shown="True" w1063 {
                frame False {
                }
                frame True {
                  n1176 = flat-sequence {
                    frame #0 {
                      n1177 = local write "Exit SC handler StMach hid"(FALSE ("Exit tester state machine hid")) -> ()
                      n1178 = local write "SC handler states hid"(SC_handler_states."initializing bus" ("SC virtual handler states")) -> ()
                    }
                    frame #1 {
                      n1179 = flat-sequence {
                        tunnel: [w1070] -> w1067
                        tunnel: [w1069] -> w1068
                        frame #0 {
                          w1069 = 0.0
                          # "These are consumed in the \"responding to sites\"\nstate when at least one handler has sites ready.  \nIt is executed only after one cycle. At that point,\nthere is at least one test period and one wait period\nto make a utilization calculation."
                          n1180 = local read "Utilization averaging"() -> (w1071:i32)
                          n1181 = Initialize Array(w1069, w1071) -> (w1070:dbl[])
                        }
                      }
                      n1182 = while {
                        shift-right: [w1079] -> _
                        shift-left: w1068 -> [w1074]
                        shift-right: [w1075] -> _
                        shift-left: w1067 -> [w1073]
                        i -> [w1072]
                        stop <- w1076 stop-if-true
                        n1183 = flat-sequence {
                          tunnel: [w1085] -> w1078
                          tunnel: [w1084] -> w1077
                          tunnel: w1074 -> [w1083]
                          tunnel: w1073 -> [w1082]
                          tunnel: [w1811] -> w1075
                          tunnel: [w1812] -> w1079
                          tunnel: w1078 -> [w1812]
                          tunnel: w1077 -> [w1811]
                          frame #0 {
                            n1184 = local read "SC handler states hid"() -> (w1081:T7)
                            n1185 = case shown="\"initializing bus\", Default" w1081 {
                              tunnel: w1083 -> [w1086 w1106 w1133 w1180 w1251 w1267 w1302 w1336 w1424 w1460 w1536 w1640 w1678 w1691 w1792 w1803]
                              tunnel: [w1087 w1107 w1134 w1181 w1252 w1268 w1301 w1335 w1421 w1459 w1535 w1639 w1677 w1690 w1791 w1802] -> w1084
                              tunnel: w1082 -> [w1087 w1107 w1134 w1181 w1252 w1268 w1301 w1335 w1423 w1459 w1535 w1639 w1677 w1690 w1791 w1802]
                              tunnel: [w1086 w1106 w1133 w1180 w1251 w1267 w1302 w1336 w1422 w1460 w1536 w1640 w1678 w1691 w1792 w1803] -> w1085
                              frame "initializing bus", Default {
                                n1186 = flat-sequence {
                                frame #0 {
                                n1187 = local write "VISA bus 0 close error"(FALSE ("VISA bus 0 close error")) -> ()
                                }
                                frame #1 {
                                w1096 = T14 1073684500 items=["Service Request"=1073684491, "Trigger"=3221168138, "Clear"=1073684493, "VXI Signal"=1073684512, "VXI/VME Interrupt"=3221168161, "VXI/VME Sysfail"=1073684509, "VXI/VME Sysreset"=1073684510, "GPIB CIC"=1073684498, "GPIB Talk"=1073684499, "GPIB Listen"=1073684500, "PXI Interrupt"=1073684514, "Serial Break"=1073684515, "Serial TermChar"=1073684516, "Serial CTS"=1073684521, "Serial DSR"=1073684522, "Serial DCD"=1073684524, "Serial RI"=1073684526, "Serial Character"=1073684533, "USB Interrupt"=1073684535, "All Enabled"=1073709055] ("Event Type")
                                n1188 = local read "SentCtrl listens to tester at"() -> (w1093:refnum<visa-resource-name>)
                                n1189 = local read "GPIB wait timeout hid"() -> (w1091:u32)
                                n1190 = VISA Open(VISA resource name=w1093) -> (VISA resource name=w1098:refnum<visa-resource-name>, error out=w1097:errorcluster)  [unwired: 1 in, 3 out]
                                n1191 = Unbundle By Name(w1097) -> ()  [unwired: 1 out]
                                n1192 = property class="GPIB BoardInterface"(reference=w1098, error in=w1097, "General Settings:Timeout Value"=w1091) -> (reference out=w1095:refnum<visa-resource-name>, error out=w1094:errorcluster)
                                n1193 = VISA Enable Event(8:w1094, 10:w1096, 11:w1095) -> (0:w1090:errorcluster, 3:→"VISA bus 0 resource name out hid":refnum<visa-resource-name>)  [unwired: 1 out]
                                "VISA bus 0 error out hid" <- w1090
                                n1194 = Unbundle By Name(w1090) -> ("status"=w1089:bool)
                                n1195 = local write "VISA bus 0 open error"(w1089) -> ()
                                }
                                frame #2 {
                                n1196 = Concatenate Strings("Bus 0 initializing " ("string"), "\r\n") -> (w1100:string)
                                n1197 = local write "GPIB Bus 0 traffic"(w1100) -> ()
                                }
                                frame #3 {
                                n1198 = local write "Exit SC handler StMach hid"(FALSE ("Exit tester state machine hid")) -> ()
                                }
                                frame #4 {
                                n1199 = local read "Tester Handler Config"() -> (w1103:T2)
                                n1200 = case shown="\"Seiko-Epson NS6040\"" w1103 {
                                frame "Multitest", Default {
                                n1201 = local write "SC handler states hid"(SC_handler_states."waiting on event" ("SC Test Interface States")) -> ()
                                }
                                frame "Seiko-Epson NS6040" {
                                n1202 = local write "SC handler states hid"(SC_handler_states."waiting on serial poll" ("SC Test Interface States")) -> ()
                                }
                                }
                                }
                                }
                              }
                              frame "waiting on event" {
                                n1203 = flat-sequence {
                                frame #0 {
                                n1204 = local read "GPIB Bus 0 traffic"() -> (w1108:string)
                                n1205 = Concatenate Strings(w1108, "\r\n", "Bus 0 waiting on event" ("string")) -> (w1111:string)
                                n1206 = local write "GPIB Bus 0 traffic"(w1111) -> ()
                                }
                                frame #1 {
                                n1207 = local read "VISA bus 0 resource name out hid"() -> (w1121:refnum<visa-resource-name>)
                                n1208 = local read "VISA bus 0 error out hid"() -> (w1120:errorcluster)
                                n1209 = local read "GPIB wait timeout hid"() -> (w1119:u32)
                                n1210 = VISA Wait on Event(7:w1119, 8:w1120, 11:w1121) -> (0:w1112:errorcluster, 3:w1113:refnum<visa-resource-name>)  [unwired: 2 in, 2 out]
                                n1211 = local write "VISA bus 0 resource name out hid"(w1113) -> ()
                                n1212 = local write "VISA bus 0 error out hid"(w1112) -> ()
                                n1213 = Unbundle By Name(w1112) -> ("status"=w1116:bool)
                                n1214 = Unbundle By Name(w1112) -> ("code"=w1118:i32)
                                n1215 = Equal?(x=w1118, y=-1073807339) -> (x = y?=w1115:bool)
                                n1216 = Or(x=w1116, y=w1115) -> (x .or. y?=w1114:bool)
                                n1217 = case shown="True" w1114 {
                                tunnel: w1113 -> [_ w1124]
                                tunnel: w1112 -> [_ w1123]
                                frame False {
                                n1218 = local write "SC handler states hid"(SC_handler_states."reading" ("SC Test Interface States")) -> ()
                                }
                                frame True {
                                n1219 = flat-sequence {
                                tunnel: w1124 -> [w1128]
                                tunnel: w1123 -> [w1127]
                                frame #0 {
                                n1220 = VISA Close(VISA resource name=w1128, error in (no error)=w1127) -> (error out=w1126:errorcluster)
                                n1221 = Unbundle By Name(w1126) -> ("status"=w1125:bool)
                                n1222 = local write "VISA bus 0 close error"(w1125) -> ()
                                }
                                frame #1 {
                                n1223 = Concatenate Strings("GPIB bus 0 error or time out waiting on event,\nclosing Bus 0 and re-initializing." ("string"), "\r\n") -> (w1131:string)
                                n1224 = local write "GPIB Bus 0 traffic"(w1131) -> ()
                                }
                                frame #2 {
                                n1225 = local write "SC handler states hid"(SC_handler_states."initializing bus" ("SC Test Interface States")) -> ()
                                }
                                }
                                }
                                }
                                }
                                }
                              }
                              frame "waiting on serial poll" {
                                n1226 = flat-sequence {
                                frame #0 {
